vi "Is Child Alias.vi"(7 "Actor in":refnum<class "Actor.lvclass">, 10 "Alias":string) -> (1 "Found":bool, 2 "Child Attributes":T1)   [LabVIEW 2020, in "jettl.lvlib" / "Actor Specific.lvlib"]
uses:
  Actor Specific.lvlib
  Actor/Actor.lvclass
  Msg/Msg.lvclass
  Msgs.ctl
  jettl.lvlib
  Unified Layer.ctl
  Actor Attributes.ctl
  Msg Input/Msg Input.lvclass
  Msg Output/Msg Output.lvclass
  Relation.ctl
  Teller.ctl
  Msg Attributes.ctl
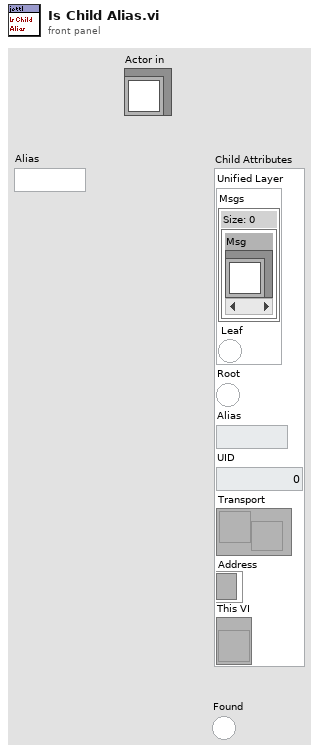
[diagram p1: front panel]
types:
  T1 = typedef "jettl.lvlib/Actor Attributes.ctl" = cluster{"Unified Layer":T2, "Root":bool, "Alias":string, "UID":i32, "Transport":refnum<user-event>, "Address":refnum<event-registration>, "This VI":refnum<vi>}
  T2 = typedef "jettl.lvlib/Unified Layer.ctl" = cluster{"Msgs":T3, "Leaf":bool}
  T3 = typedef "jettl.lvlib/Msgs.ctl" = set{refnum<class "Msg.lvclass">}
  T4 = typedef "jettl.lvlib/Child Actor Attributes.ctl" = map{string, T1}
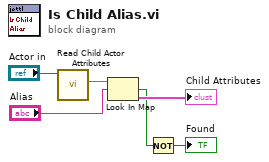
[diagram p0: block diagram]
diagram:
  n1 = call-dynamic "Read Child Actor Attributes.vi"("Actor in"="Actor in") -> ("Child Actor Attributes"=w1:T4)  [unwired: 10 in]
  n2 = Look In Map(map=w1, key="Alias") -> (key not found?=w3:bool, value=→"Child Attributes":T1)  [unwired: 1 in]
  n3 = Not(x=w3) -> (.not. x?=→"Found":bool)
